vi "update.path.vi"(8 "error in":errorcluster, 11 "Run":refnum<class "Run.lvclass">) -> (0 "error out":errorcluster, 2 "path":string, 3 "Run Out":refnum<class "Run.lvclass">)   [LabVIEW 2020, in "Run.lvclass"]
uses:
  Run.lvclass
  Run.lvclass/Run.ctl
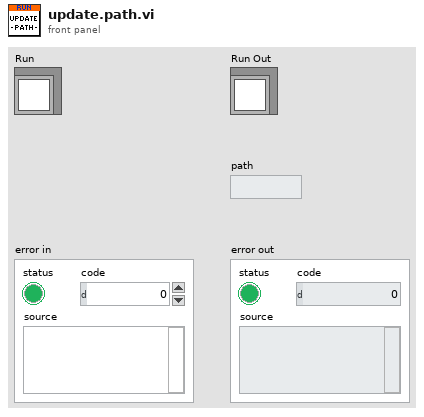
[diagram p1: front panel]
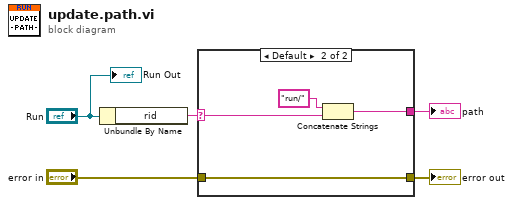
[diagram p0: block diagram]
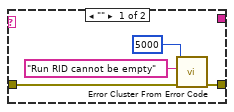
[diagram p2: hidden frame]
diagram:
  n1 = Unbundle By Name("Run") -> ("rid"=w2:string)
  n2 = case shown="Default" w2 {
    selector: w2 -> [_ w12]
    tunnel: [_ w11] -> w5
    tunnel: "error in" -> [w9 w10]
    tunnel: [w7 w10] -> w3
    frame "" {
      n3 = call <vilib>:"Error Cluster From Error Code.vi"("error in (no error)"=w9, "error message (\"\")"="Run RID cannot be empty" ("error message (\"\")"), "error code (0)"=5000) -> ("error out"=w7:errorcluster)  [unwired: 6 in]
    }
    frame Default {
      n4 = Concatenate Strings("run/" ("path"), w12) -> (w11:string)
    }
  }
  "path" <- w5
  "error out" <- w3
  "Run Out" <- "Run"
